vi "IsErrorCluster_2.vi"(1 "UseLV2011Compatibility":bool=TRUE, 4 "Data Types":string[](array[string]), 5 "Dirs":T1[](array[typedef])) -> (0 "Dirs Out":T1[](array[typedef]))   [LabVIEW 2020]
uses:
  <vilib>/AppBuilder/IOStatus.ctl
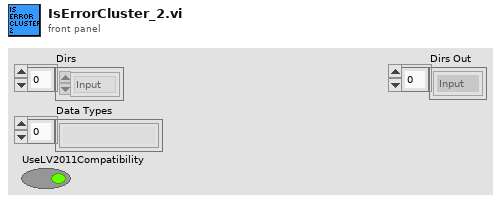
[diagram p1: front panel]
types:
  T1 = typedef "IOStatus.ctl" = enum16{"Input", "Output", "Input/Output", "InputDeleted", "OutputDeleted", "IODeleted", "ErrorClusterIn", "ErrorClusterOut"}
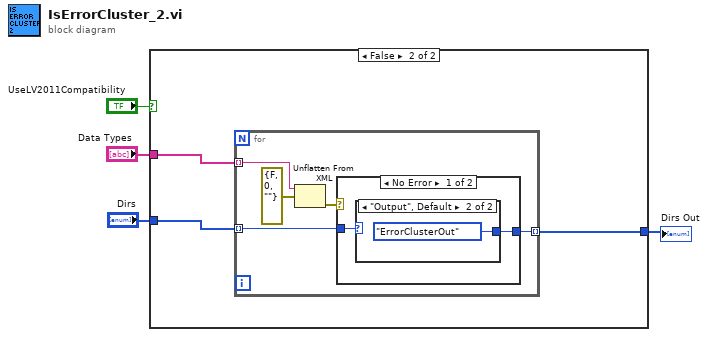
[diagram p0: block diagram]
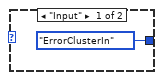
[diagram p3: hidden frame]
diagram:
  n1 = case shown="False" "UseLV2011Compatibility" {
    tunnel: "Dirs" -> [w5 w7]
    tunnel: "Data Types" -> [_ w8]
    tunnel: [w5 w6] -> w1
    frame True {
    }
    frame False {
      n2 = for {
        tunnel: w8 -> [w13] mode=indexing
        tunnel: w7 -> [w10] mode=indexing
        tunnel: [w9] -> w6 mode=indexing
        n3 = Unflatten From XML(xml string=w13, type=errorcluster {"status"=FALSE, "code"=0, "source"=""} ("error constant")) -> (error out=w11:errorcluster)  [unwired: 1 in, 1 out]
        n4 = case shown="No Error" w11 {
          tunnel: w10 -> [w15 w18]
          tunnel: [w14 w18] -> w9
          frame No Error {
            n5 = case shown="\"Output\", Default" w15 {
              tunnel: [IOStatus."ErrorClusterIn" ("dir") IOStatus."ErrorClusterOut" ("dir")] -> w14
              frame "Input" {
              }
              frame "Output", Default {
              }
            }
          }
          frame Error {
          }
        }
      }
    }
  }
  "Dirs Out" <- w1
